vi "Decorate.vi"(10 "Event":refnum<class "Event.lvclass">, 11 "Template Event in":refnum<class "Template Event.lvclass">) -> (3 "Template Event out":refnum<class "Template Event.lvclass">)   [LabVIEW 2021, in "_Template.lvlib" / "Templates.lvlib" / "Template Event.lvlib" / "Template Event.lvclass"]
uses:
  Template Event.lvclass
  <vilib>/jettl/jettl/jettl/Event/Event.lvclass
  Template Event.lvclass/Template Event.ctl
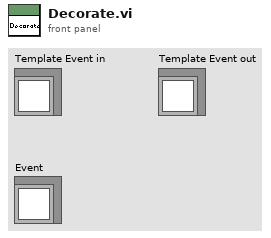
[diagram p1: front panel]
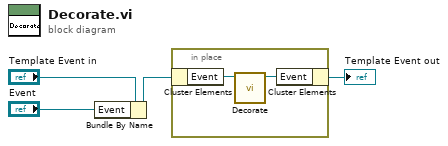
[diagram p0: block diagram]
diagram:
  n1 = Bundle By Name(cluster="Template Event in", "Event"="Event") -> (w2:refnum<class "Template Event.lvclass">)
  n2 = in-place {
    n3 = in-place-cluster #1(w2) -> ("Event"=w6:refnum<class "Event.lvclass">)
    n4 = call-dynamic "Decorate.vi"("Event in"=w6) -> ("Event out"=w5:refnum<class "Event.lvclass">)  [unwired: 10 in]
    n5 = in-place-cluster #1("Event"=w5) -> (→"Template Event out":refnum<class "Template Event.lvclass">)
  }
